vi "setPlotName.vi"(8 "reference":refnum<vi>, 10 "Array":string[][](array[string]), 11 "WaveformGraph in":refnum<vi>) -> ()   [LabVIEW 2018]
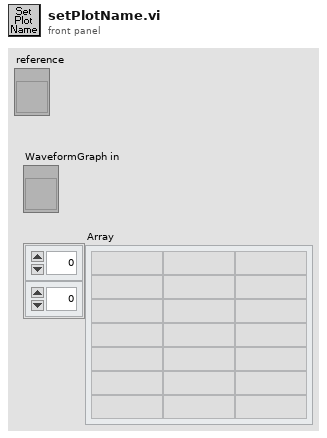
[diagram p1: front panel]
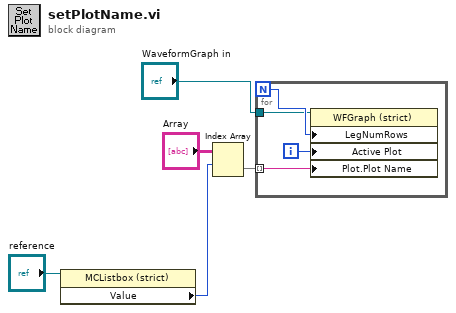
[diagram p0: block diagram]
diagram:
  n1 = property on="Property Node" class="MCListbox (strict)"(reference="reference") -> ("Value"=w1:i32)  [unwired: 1 in, 2 out]
  n2 = Index Array(array="Array", index (row)=w1) -> (element=w3:string[])  [unwired: 1 in]
  n3 = for {
    N -> [w8]
    tunnel: w3 -> [w7] mode=indexing
    tunnel: "WaveformGraph in" -> [w6]
    i -> [w9]
    n4 = property on="Property Node" class="WFGraph (strict)"(reference=w6, "LegNumRows"=w8, "Active Plot"=w9, "Plot.Plot Name"=w7) -> ()  [unwired: 1 in, 2 out]
  }
